vi "Buffer Storage Status.vi"(8 "error in (no error)":errorcluster, 11 "VISA resource name":refnum<visa-resource-name>) -> (0 "error out":errorcluster, 1 "Number of Stored Readings":string, 2 "Points Remaining":string, 3 "VISA resource name out":refnum<visa-resource-name>, 4 "Operation Complete":bool)   [LabVIEW 2015, in "IT8900A-E.lvlib"]
doc: "This command is used to read the state of the storage.After sending the command and making the load dialog, two comma-separated values are sent to the computer.The first interval indicates how many bits of the memory are available, and the second indicates how many bits are retained for the memory reading."
uses:
  <instrlib>/IT8900/IT8900A-E.lvlib
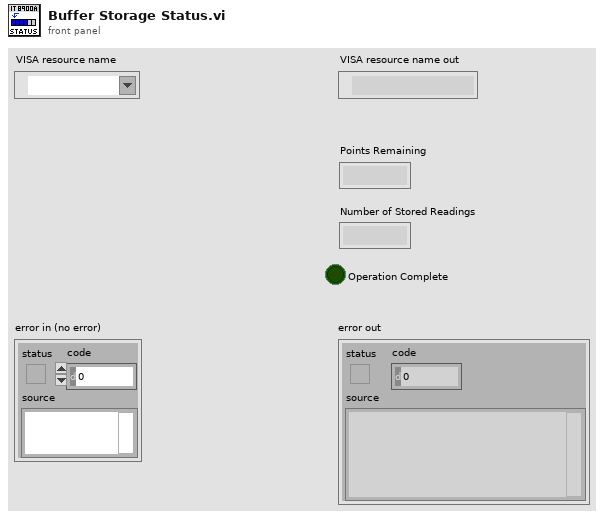
[diagram p1: front panel]
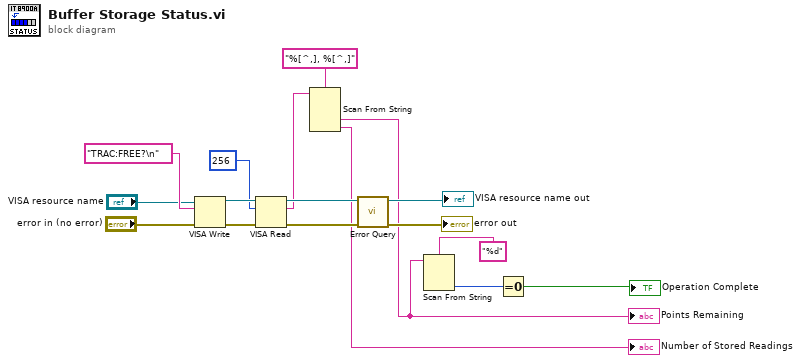
[diagram p0: block diagram]
diagram:
  n1 = VISA Write(VISA resource name="VISA resource name", write buffer="TRAC:FREE?\n", error in (no error)="error in (no error)") -> (VISA resource name out=w13:refnum<visa-resource-name>, error out=w14:errorcluster)  [unwired: 1 out]
  n2 = VISA Read(VISA resource name=w13, byte count=256, error in (no error)=w14) -> (VISA resource name out=w9:refnum<visa-resource-name>, read buffer=w7:string, error out=w8:errorcluster)  [unwired: 1 out]
  n3 = Scan From String(format string="%[^,], %[^,]", input string=w7) -> (output 1=w1:string, output 2=→"Number of Stored Readings":string)  [unwired: 4 in, 3 out]
  "Points Remaining" <- w1
  n4 = call <instrlib>:"Error Query.vi"("error in (no error)"=w8, "VISA resource name"=w9) -> ("error out"=→"error out":errorcluster, "VISA resource name out"=→"VISA resource name out":refnum<visa-resource-name>)  [unwired: 6 in, 2 out]
  n5 = Scan From String(format string="%d", input string=w1) -> (output 1=w2:i32)  [unwired: 3 in, 3 out]
  n6 = Equal To 0?(x=w2) -> (x = 0?=→"Operation Complete":bool)
